vi "Read next.vi"(8 "error in (no error)":errorcluster, 11 "NodeType in":refnum<class "IDoublyNode.lvclass">) -> (0 "error out":errorcluster, 2 "next":refnum<data-value>, 3 "NodeType out":refnum<class "IDoublyNode.lvclass">)   [LabVIEW 2021, in "IDoublyNode.lvclass"]
uses:
  IDoublyNode.lvclass
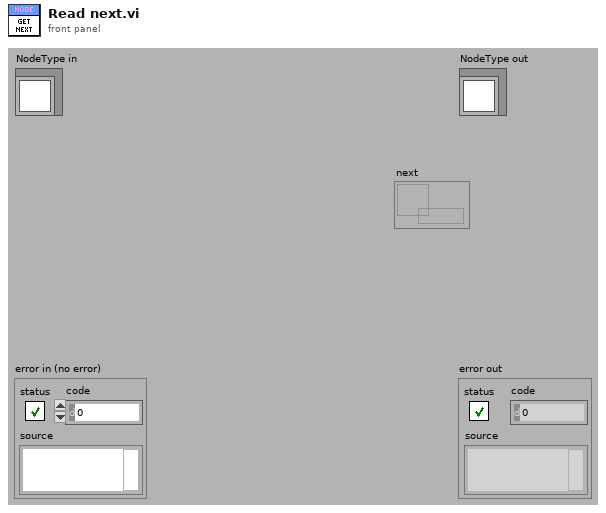
[diagram p1: front panel]
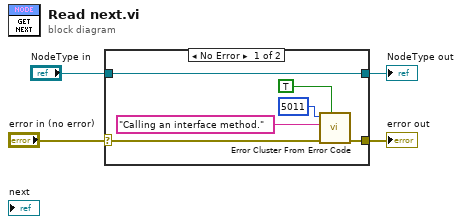
[diagram p0: block diagram]
diagram:
  n1 = case shown="No Error" "error in (no error)" {
    selector: "error in (no error)" -> [w6 w12]
    tunnel: [w5 w12] -> w3
    tunnel: [w10 w11] -> w1
    tunnel: "NodeType in" -> [w10 w11]
    frame No Error {
      n2 = call <vilib>:"Error Cluster From Error Code.vi"("show call chain? (False)"=TRUE, "error in (no error)"=w6, "error message (\"\")"="Calling an interface method." ("error message (\"\")"), "error code (0)"=5011) -> ("error out"=w5:errorcluster)  [unwired: 5 in]
    }
    frame Error {
    }
  }
  "error out" <- w3
  "NodeType out" <- w1
